vi "Receive Message.vi"(6 "priority":i32, 10 "ActorStateMachine in":refnum<class "ActorStateMachine.lvclass">, 11 "Message in":refnum<class "Message.lvclass">) -> (0 "error out":errorcluster, 2 "Actor out":refnum<class "Actor.lvclass">)   [LabVIEW 2021, in "ActorStateMachine.lvlib" / "ActorStateMachine.lvclass"]
doc: "This VI should be overriden ONLY if you are creating a proxy actor for remote transmission. If you are, override this VI to transmit the received message to a new destination, maintaining the given priority."
uses:
  ActorStateMachine.lvclass
  <vilib>/ActorFramework/Message/Message.lvclass
  <vilib>/ActorFramework/Actor/Actor.lvclass
  C:/Program Files (x86)/National Instruments/LabVIEW 2021/vi.lib/ActorFramework/Actor/Actor.lvclass
  ActorStateMachine.lvclass/ActorStateMachine.ctl
  <vilib>/ActorFramework/Stop Msg/Stop Msg.lvclass
  C:/Program Files (x86)/National Instruments/LabVIEW 2021/vi.lib/ActorFramework/Message/Message.lvclass
  <vilib>/ActorFramework/LastAck/Last Ack.lvclass
  AsmEventMessage/AsmEventMessage.lvclass
  AsmSettingsMessage/AsmSettingsMessage.lvclass
  D:/_uliarczj/_sandbox/SWTest/Utilities/LabVIEW/ActorStateMachine/Source/ActorStateMachine/AsmMessage/AsmMessage.lvclass
  D:/_uliarczj/_sandbox/SWTest/Utilities/LabVIEW/ActorStateMachine/Source/ActorStateMachine/AsmSettingsMessage/AsmSettingsMessage.lvclass
  D:/_uliarczj/_sandbox/SWTest/Utilities/LabVIEW/ActorStateMachine/Source/ActorStateMachine/AsmEventMessage/AsmEventMessage.lvclass
  C:/Program Files (x86)/National Instruments/LabVIEW 2021/vi.lib/ActorFramework/Stop Msg/Stop Msg.lvclass
  C:/Program Files (x86)/National Instruments/LabVIEW 2021/vi.lib/ActorFramework/LastAck/Last Ack.lvclass
  D:/_uliarczj/_sandbox/SWTest/Utilities/LabVIEW/ActorStateMachine/Source/ActorStateMachine/ActorStateMachine/ActorStateMachine.lvclass
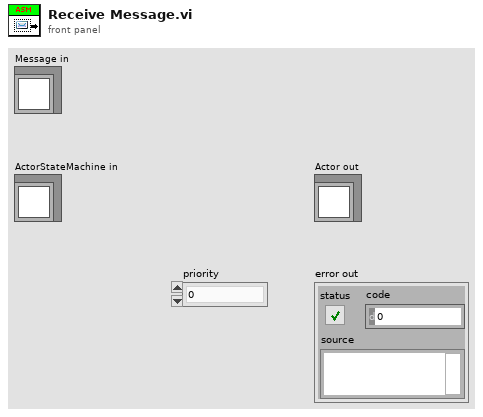
[diagram p1: front panel]
types:
  T1 = typedef "ActorStateMachine.lvlib/ActorStateMachine.lvclass/_ASM.State.ctl" = enum16{"Boom", "Pre-Init", "Init", "Post-Init", "Pre-Reset", "Reset", "Post-Reset", "Pre-Config", "Config", "Post-Config", "Pre-Ready", "Ready", "Post-Ready", "Pre-Running", "Running", "Next", "Post-Running", "Break", "Fail", "Crash", "Shutdown", "Doom"}
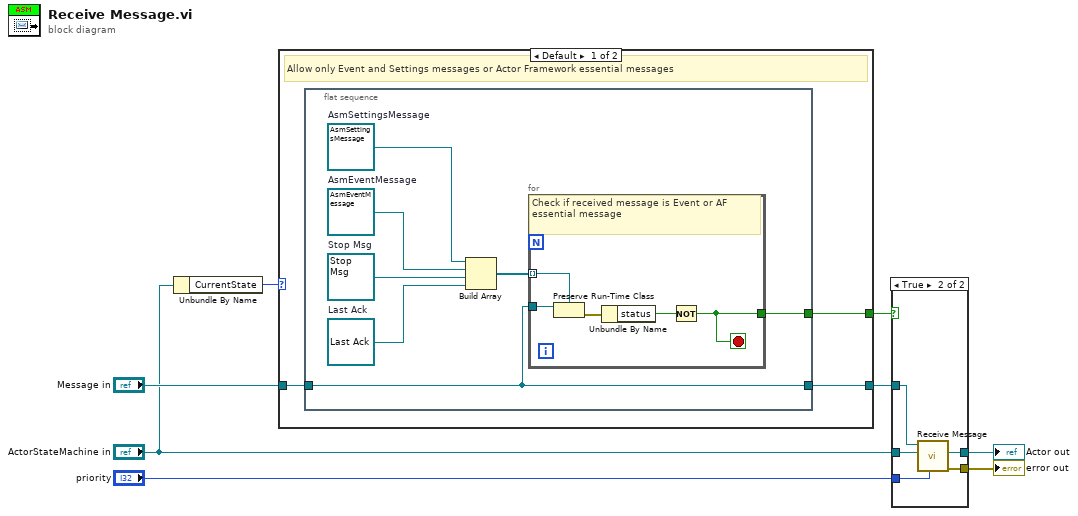
[diagram p0: block diagram]
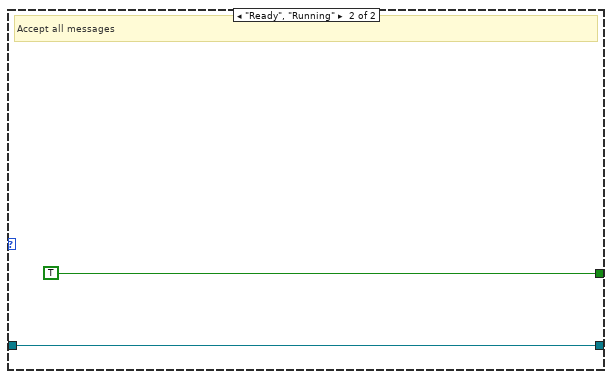
[diagram p3: hidden frame]
diagram:
  n1 = Unbundle By Name("ActorStateMachine in") -> ("CurrentState"=w1:T1)
  n2 = case shown="Default" w1 {
    tunnel: "Message in" -> [w10 w24]
    tunnel: [w11 TRUE] -> w5
    tunnel: [w9 w24] -> w3
    frame Default {
      # "Allow only Event and Settings messages or Actor Framework essential messages"
      n3 = flat-sequence {
        tunnel: [w14] -> w11
        tunnel: w10 -> [w12]
        tunnel: [w12] -> w9
        frame #0 {
          w13 = refnum<class "AsmSettingsMessage.lvclass"> refnum  # AsmSettingsMessage
          w18 = refnum<class "AsmEventMessage.lvclass"> refnum  # AsmEventMessage
          w16 = refnum<class "Last Ack.lvclass"> refnum  # Last Ack
          w17 = refnum<class "Stop Msg.lvclass"> refnum  # Stop Msg
          n4 = Build Array(w13, w18, w17, w16) -> (w15:refnum<class "Message.lvclass">[])
          n5 = for {
            tunnel: w15 -> [w23] mode=indexing
            tunnel: w12 -> [w22]
            tunnel: [w19] -> w14
            stop <- w19 stop-if-true
            # "Check if received message is Event or AF essential message"
            n6 = Preserve Run-Time Class(object in=w22, 2:w23) -> (error out=w21:errorcluster)  [unwired: 1 in, 1 out]
            n7 = Unbundle By Name(w21) -> ("status"=w20:bool)
            n8 = Not(x=w20) -> (.not. x?=w19:bool)
          }
        }
      }
    }
    frame "Ready", "Running" {
      # "Accept all messages"
    }
  }
  n9 = case shown="True" w5 {
    tunnel: w3 -> [_ w31]
    tunnel: "ActorStateMachine in" -> [w26 w30]
    tunnel: "priority" -> [_ w29]
    tunnel: [_ w28] -> w7
    tunnel: [w26 w27] -> w6
    frame False {
    }
    frame True {
      n10 = call-parent "Receive Message.vi"("priority"=w29, "Actor in"=w30, "Message in"=w31) -> ("error out"=w28:errorcluster, "Actor out"=w27:refnum<class "Actor.lvclass">)  [unwired: 7 in]
    }
  }
  "error out" <- w7
  "Actor out" <- w6
